vi "Get Next Win Msg.vi"(4 "error in (no error)":errorcluster, 7 "win msg queue":T1) -> (0 "error out":errorcluster, 1 "Sent":bool, 2 "Message":T2 {"Msg" format="%.0x"; "hWnd" format="%.0x"}, 3 "win msg queue out":T1)   [LabVIEW 2011]
doc: "Removes the next message from the windows message queue and returns it. This should only be used after a call to Windows Message Queue Size.vi is used to determine how many messages are available in the queue.\n\nParameters:\nwin msg queue: the queue from which to remove the message.\n\nMessage: the message returned. The cluster is of the same format as the Windows MSG structure and contains the following information:\n hWnd: the handle of the window to which the message was posted\n message: the message\n wParam: the wParam parameter. Specific meaning depends on message.\n lParam: the lParam parameter. Specific meaning depends on message.\n time: system time at which the message was posted\n point: point cluster contain mouse positon in screen \n coordinates at the time of message posting\n\nSent: returns true if the message was sent to the window (via a call to SendMessage) or false if the message was posted (via PostMessage). Note: messages that are sent will not have valid time or point parameters.\n\nErrors:\n6751: Not a valid windows message queue.\n6752: No elements in queue."
uses:
  Win Msg Q RefNum.ctl
  Win Msg.ctl
  lvwinmsg.dll
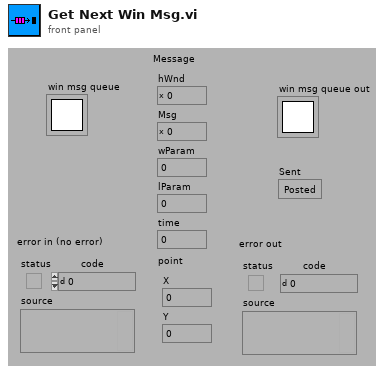
[diagram p1: front panel]
types:
  T1 = typedef "Win Msg Q RefNum.ctl" = refnum<k1>
  T2 = typedef "Win Msg.ctl" = cluster{"hWnd":u32, "Msg":u32, "wParam":u32, "lParam":i32, "time":u32, "point":cluster{"X":i32, "Y":i32}}
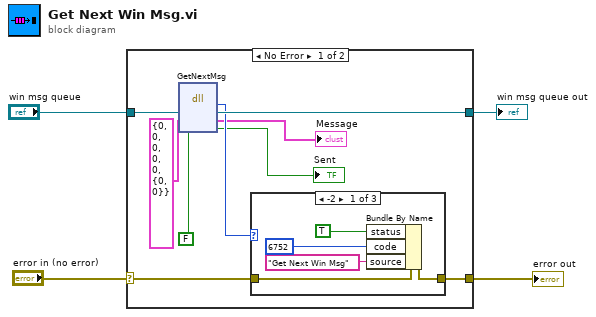
[diagram p0: block diagram]
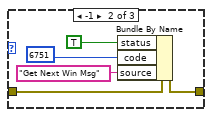
[diagram p2: hidden frame]
diagram:
  n1 = case shown="No Error" "error in (no error)" {
    selector: "error in (no error)" -> [w7 w25]
    tunnel: "win msg queue" -> [w12 w26]
    tunnel: [w13 w25] -> w3
    tunnel: [w10 w26] -> w2
    frame No Error {
      n2 = dll-call lib="C:/Development/SI.LIB/WIN32/WinMSGQ/lvwinmsg.dll" fn="GetNextMsg"("win msg queue"=w12, "Input Value"=T2 {"hWnd"=0, "Msg"=0, "wParam"=0, "lParam"=0, "time"=0, "point"={"X"=0, "Y"=0}}, "output param"=FALSE) -> (w9:i32, "win msg queue"=w10:T1, "Input Value"=→"Message":T2, "output param"=→"Sent":bool)  [unwired: 3 in, 2 out]
      n3 = case shown="-2" w9 {
        tunnel: w7 -> [w18 w21 w24]
        tunnel: [w17 w20 w24] -> w13
        frame -2 {
          n4 = Bundle By Name(cluster=w18, "status"=TRUE, "code"=6752 ("Error Code"), "source"="Get Next Win Msg") -> (w17:errorcluster)
        }
        frame -1 {
          n5 = Bundle By Name(cluster=w21, "status"=TRUE, "code"=6751 ("Error Code"), "source"="Get Next Win Msg") -> (w20:errorcluster)
        }
        frame 1, Default {
        }
      }
    }
    frame Error {
    }
  }
  "error out" <- w3
  "win msg queue out" <- w2
